vi "Sellmeier.vi"() -> ()   [LabVIEW 2018]
uses:
  <vilib>/express/express arith-compare/Formula/XNode/ExpressFormulaBlockNode.xnode
panel:
  out "SHG theta":dbl
  out "lam_idler(o) (nm)":dbl
  out "lam_shg(e) (nm)":dbl
  in  "lam_signal(nm)":dbl
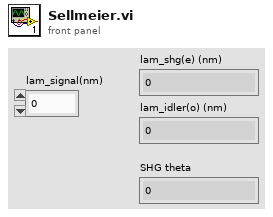
[diagram p1: front panel]
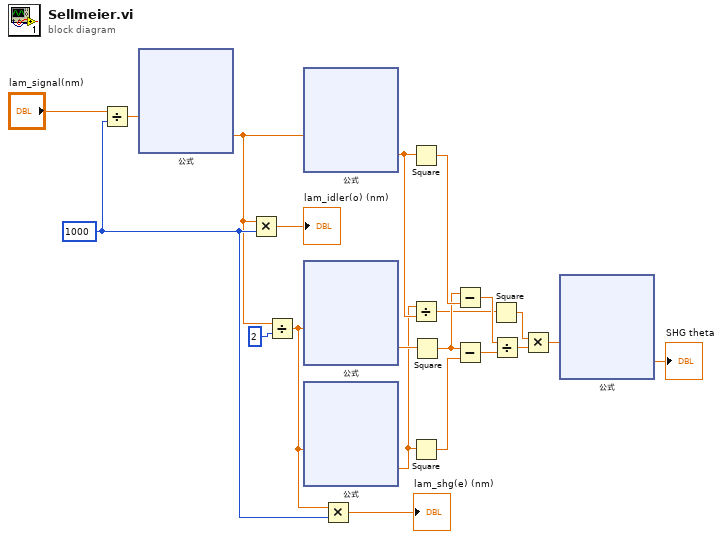
[diagram p0: block diagram]
diagram:
  w6 = 1000
  n1 = Divide(x="lam_signal(nm)", y=w6) -> (x/y=w5:dbl)
  n2 = xnode "公式"("lam"=w5) -> ("结果"=w4:dbl)  [unwired: 1 in, 1 out]
  n3 = Multiply(x=w4, y=w6) -> (x*y=→"lam_idler(o) (nm)":dbl)
  n4 = Divide(x=w4, y=2) -> (x/y=w1:dbl)
  n5 = xnode "公式"("lam"=w4) -> ("结果"=w14:dbl)  [unwired: 1 in, 1 out]
  n6 = xnode "公式"("lam"=w1) -> ("结果"=w18:dbl)  [unwired: 1 in, 1 out]
  n7 = xnode "公式"("lam"=w1) -> ("结果"=w10:dbl)  [unwired: 1 in, 1 out]
  n8 = Multiply(x=w1, y=w6) -> (x*y=→"lam_shg(e) (nm)":dbl)
  n9 = Square(x=w14) -> (x^2=w19:dbl)
  n10 = Divide(x=w10, y=w14) -> (x/y=w12:dbl)
  n11 = Square(x=w10) -> (x^2=w11:dbl)
  n12 = Square(x=w18) -> (x^2=w13:dbl)
  n13 = Subtract(x=w13, y=w19) -> (x-y=w17:dbl)
  n14 = Subtract(x=w13, y=w11) -> (x-y=w16:dbl)
  n15 = Square(x=w12) -> (x^2=w20:dbl)
  n16 = Divide(x=w17, y=w16) -> (x/y=w15:dbl)
  n17 = Multiply(x=w20, y=w15) -> (x*y=w8:dbl)
  n18 = xnode "公式"("X1"=w8) -> ("结果"=→"SHG theta":dbl)  [unwired: 1 in, 1 out]
